vi "PracticalUnderstandingWithDb.vi"() -> ()   [LabVIEW 2019]
uses:
  <vilib>/addons/database/Connection.llb/DB Tools Open Connec (String).vi
  <vilib>/addons/database/NI_Database_API.lvlib
panel:
  out "Data from Table":variant[][](array[variant])
  out "error out":errorcluster
  # "Serial No"
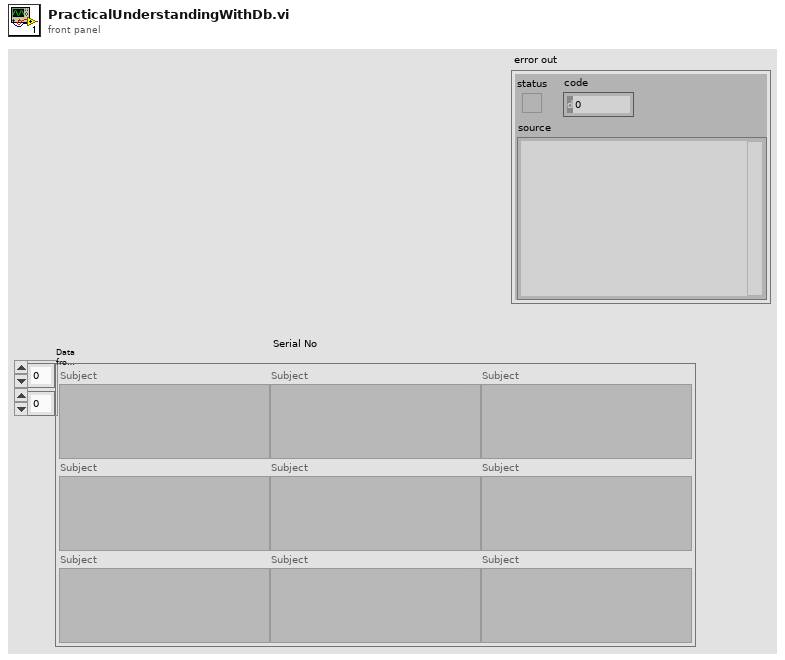
[diagram p1: front panel]
types:
  T1 = typedef "NI_Database_API.lvlib/Conn ObjectReference.ctl" = refnum<k1>
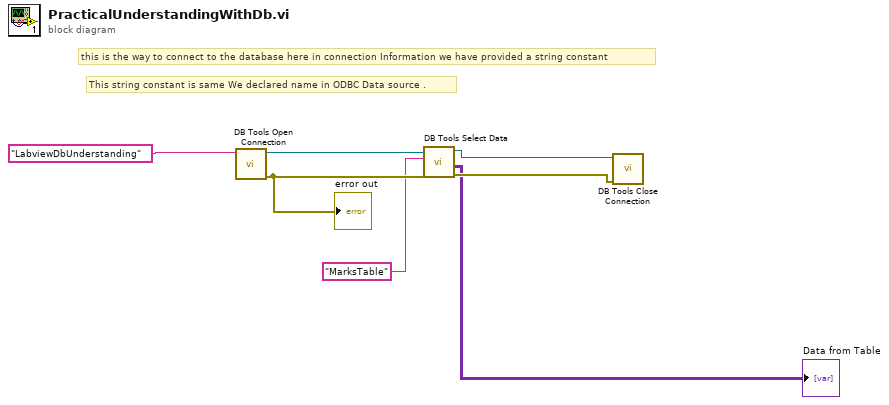
[diagram p0: block diagram]
diagram:
  # "This string constant is same We declared name in ODBC Data source ."
  # "this is the way to connect to the database here in connection Information we have provided a string constant"
  n1 = call-poly <vilib>:"DB Tools Open Connection.vi"("connection information"="LabviewDbUnderstanding") -> ("error out"=w5:errorcluster, "connection reference"=w6:T1)  [unwired: 7 in]
  "error out" <- w5
  n2 = call <vilib>:"DB Tools Select Data.vi"("error in (no error)"=w5, "table"="MarksTable", "connection reference"=w6) -> ("error out"=w2:errorcluster, "data"=→"Data from Table":variant[][], "connection reference out"=w3:T1)  [unwired: 3 in]
  n3 = call <vilib>:"DB Tools Close Connection.vi"("error in (no error)"=w2, "connection reference"=w3) -> ()  [unwired: 5 in, 1 out]
